vi "Read actual_play.vi"(8 "error in (no error)":errorcluster, 11 "Playbook in":refnum<class "Playbook.lvclass">) -> (0 "error out":errorcluster, 2 "Play":refnum<class "Play.lvclass">, 3 "Playbook out":refnum<class "Playbook.lvclass">)   [LabVIEW 2020, in "Playbook.lvclass"]
uses:
  Playbook.lvclass
  Play_class/Play.lvclass
  Playbook.lvclass/Playbook.ctl
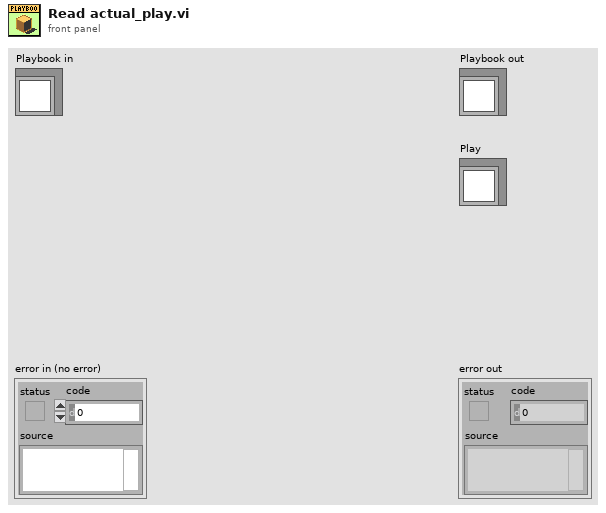
[diagram p1: front panel]
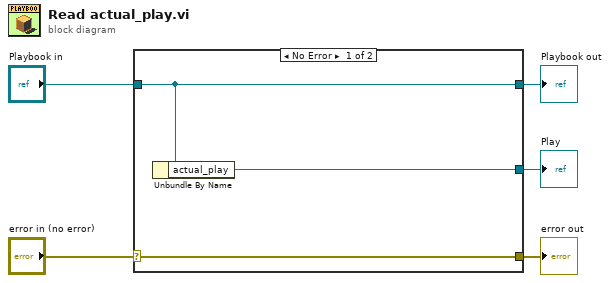
[diagram p0: block diagram]
diagram:
  n1 = case shown="No Error" "error in (no error)" {
    selector: "error in (no error)" -> [w8 w9]
    tunnel: [w8 w9] -> w4
    tunnel: [w7 w10] -> w2
    tunnel: "Playbook in" -> [w7 w10]
    tunnel: [w6 _] -> w1
    frame No Error {
      n2 = Unbundle By Name(w7) -> ("actual_play"=w6:refnum<class "Play.lvclass">)
    }
    frame Error {
    }
  }
  "error out" <- w4
  "Playbook out" <- w2
  "Play" <- w1
